vi "N simu temp.vi"(9 "Limite Minimo":dbl, 10 "Limite Maximo":dbl, 11 "Numeric":u8) -> (3 "Array":dbl[](array[numeric]))   [LabVIEW 2020]
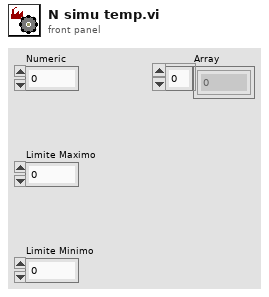
[diagram p1: front panel]
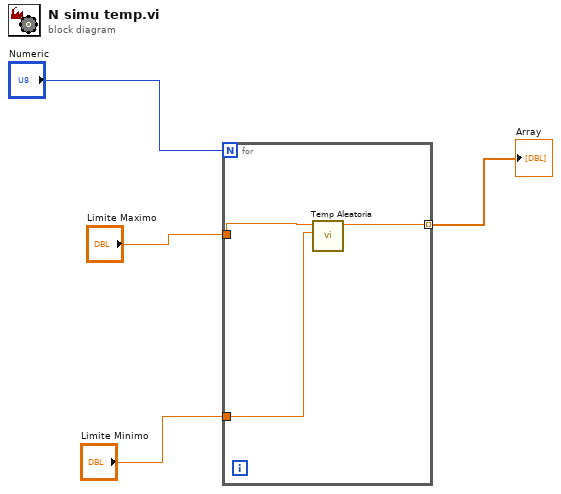
[diagram p0: block diagram]
diagram:
  n1 = for {
    N: "Numeric" -> [_]
    tunnel: "Limite Maximo" -> [w7]
    tunnel: "Limite Minimo" -> [w6]
    tunnel: [w5] -> w4 mode=indexing
    n2 = call "Temp Aleatoria.vi"("Limite Minimo"=w6, "Limite Maximo"=w7) -> ("Numeric"=w5:dbl)  [unwired: 9 in]
  }
  "Array" <- w4
